vi "Current2Grad.vi"(11 "I(A)":dbl) -> (3 "dB(mG/cm)":dbl)   [LabVIEW 2012]
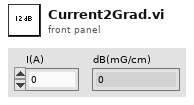
[diagram p1: front panel]
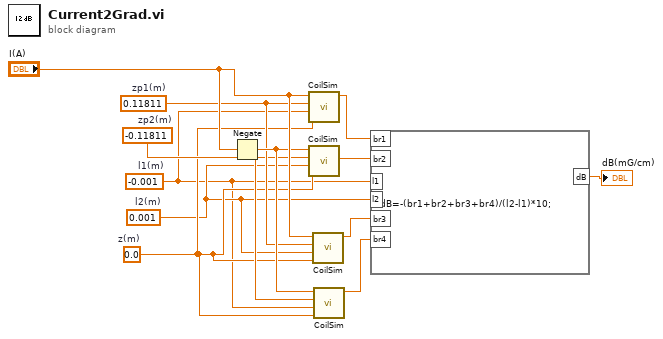
[diagram p0: block diagram]
diagram:
  w5 = 0.0  # z(m)
  w4 = 0.001  # l2(m)
  w3 = -0.001  # l1(m)
  w6 = -0.11811  # zp2(m)
  w7 = 0.11811  # zp1(m)
  n1 = Negate(x="I(A)") -> (-x=w8:dbl)
  n2 = call "CoilSim.vi"("z(m)"=w5, "x(m)"=w3, "zp(m)"=w7, "I(A)"="I(A)") -> ("Br(G)"=w12:dbl)  [unwired: 6 in, 1 out]
  n3 = call "CoilSim.vi"("z(m)"=w5, "x(m)"=w4, "zp(m)"=w6, "I(A)"=w8) -> ("Br(G)"=w11:dbl)  [unwired: 6 in, 1 out]
  n4 = call "CoilSim.vi"("z(m)"=w5, "x(m)"=w4, "zp(m)"=w7, "I(A)"="I(A)") -> ("Br(G)"=w2:dbl)  [unwired: 6 in, 1 out]
  n5 = call "CoilSim.vi"("z(m)"=w5, "x(m)"=w3, "zp(m)"=w6, "I(A)"=w8) -> ("Br(G)"=w1:dbl)  [unwired: 6 in, 1 out]
  n6 = formula code="dB=-(br1+br2+br3+br4)/(l2-l1)*10;"("br1"=w12, "br2"=w11, "l1"=w3, "l2"=w4, "br3"=w2, "br4"=w1) -> ("dB"=→"dB(mG/cm)":dbl)
